vi "RampLoop.vi"(0 "reset_ramp_x":bool, 5 "edge detected":bool, 7 "total number of ramps":i16, 9 "direction increment":i16) -> (4 "DisplacementFinished":bool, 6 "MaxNoRamp":bool, 8 "Ramp index":cluster{"ramp index":i16, "NextRamp":i16})   [LabVIEW 2016]
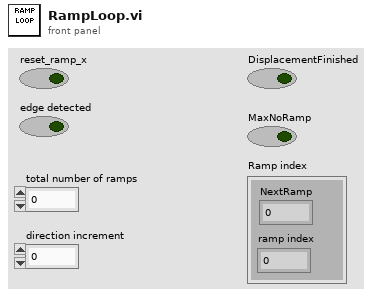
[diagram p1: front panel]
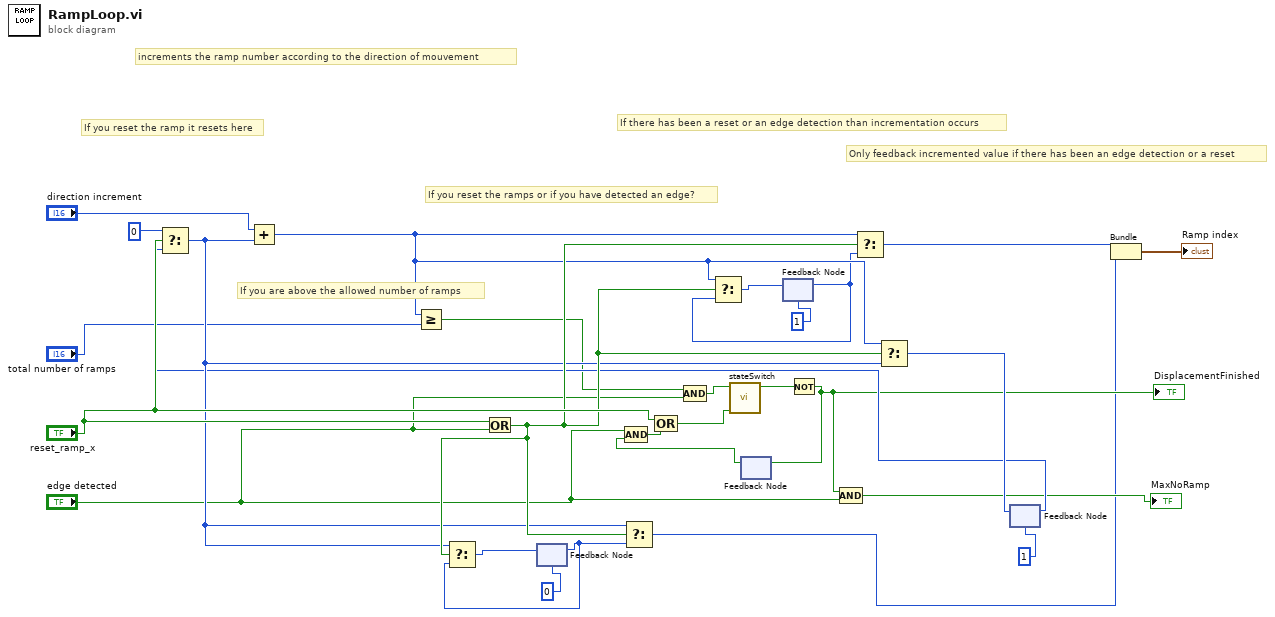
[diagram p0: block diagram]
diagram:
  # "Only feedback incremented value if there has been an edge detection or a reset"
  # "If there has been a reset or an edge detection than incrementation occurs"
  # "If you reset the ramps or if you have detected an edge?"
  # "If you are above the allowed number of ramps"
  # "If you reset the ramp it resets here"
  # "increments the ramp number according to the direction of mouvement"
  n1 = Or(x="reset_ramp_x", y="edge detected") -> (x .or. y?=w24:bool)
  n2 = feedback #1(i16 0) -> (w26:i16)
  n3 = feedback #2() -> (w11:bool)  [unwired: 1 in]
  n4 = Compound Arithmetic op=AND("edge detected", w11) -> (w10:bool)
  n5 = Compound Arithmetic op=OR("reset_ramp_x", w10) -> (w12:bool)
  n6 = feedback #3(i16 1) -> (w17:i16)
  n7 = feedback #4(i16 1) -> (w20:i16)
  n8 = Select(t=i16 0, s="reset_ramp_x", f=w20) -> (s? t:f=w23:i16)
  n9 = Add(x="direction increment", y=w23) -> (x+y=w21:i16)
  n10 = Greater Or Equal?(x=w21, y="total number of ramps") -> (x >= y?=w7:bool)
  n11 = Select(t=w23, s=w24, f=w26) -> (s? t:f=w27:i16)
  n12 = feedback-in #1(w27) -> ()
  n13 = Select(t=w23, s=w24, f=w26) -> (s? t:f=w2:i16)
  n14 = Compound Arithmetic op=AND(w7, "edge detected") -> (w8:bool)
  n15 = Select(t=w21, s=w24, f=w17) -> (s? t:f=w16:i16)
  n16 = call "stateSwitch.vi"("disable"=w12, "enable"=w8) -> ("state"=w9:bool)  [unwired: 9 in]
  n17 = feedback-in #3(w16) -> ()
  n18 = Not(x=w9) -> (.not. x?=w13:bool)
  "DisplacementFinished" <- w13
  n19 = feedback-in #2(w13) -> ()
  n20 = Compound Arithmetic op=AND(w13, "edge detected") -> (→"MaxNoRamp":bool)
  n21 = Select(t=w21, s=w24, f=w17) -> (s? t:f=w3:i16)
  n22 = Select(t=w21, s=w24, f=w23) -> (s? t:f=w22:i16)
  n23 = feedback-in #4(w22) -> ()
  n24 = Bundle(w3, w2) -> (→"Ramp index":cluster{i16, i16})  [unwired: 1 in]
